vi "Resolve IP.vi"(7 "Host to Ping":string, 8 "Error In":errorcluster) -> (0 "Error Out":errorcluster, 3 "Resolved IP":u32 format="%x")   [LabVIEW 2018]
uses:
  Instance           1 18Saved   Resolve IP .vi
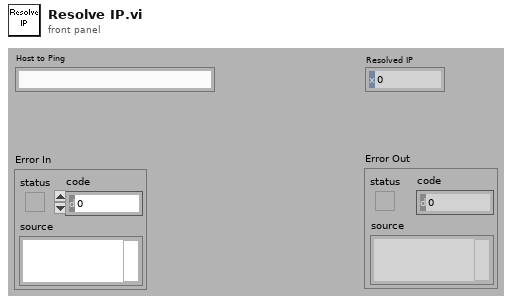
[diagram p1: front panel]
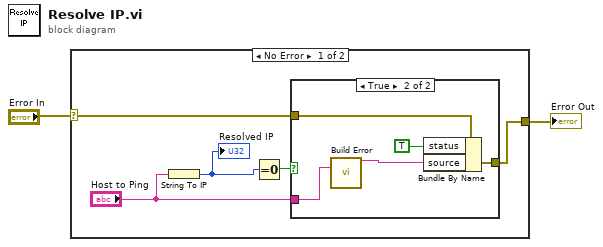
[diagram p0: block diagram]
diagram:
  n1 = case shown="No Error" "Error In" {
    selector: "Error In" -> [w7 w14]
    tunnel: [w6 w14] -> w1
    frame No Error {
      n2 = String To IP(1:"Host to Ping") -> (0:w4:u32)
      "Resolved IP" <- w4
      n3 = Equal To 0?(x=w4) -> (x = 0?=w5:bool)
      n4 = case shown="True" w5 {
        tunnel: [w8 w13] -> w6
        tunnel: "Host to Ping" -> [_ w9]
        tunnel: w7 -> [w8 w11]
        frame False {
          # "IP was resolved without error"
        }
        frame True {
          n5 = call "Build Error"("host"=w9) -> ("Result"=w10:string)  [unwired: 13 in, 1 out]
          n6 = Bundle By Name(cluster=w11, "status"=TRUE, "source"=w10) -> (w13:errorcluster)
        }
      }
    }
    frame Error {
    }
  }
  "Error Out" <- w1
